vi "一体站流程自动启动.vi"(11 "参数":T1) -> ()   [LabVIEW 2016, in "PLC.lvlib"]
uses:
  PLC.lvlib
panel:
  out "s? t:f":enum16{"初始化", "采配水启动", "仪器操作", "反冲洗", "结束"}(ring)
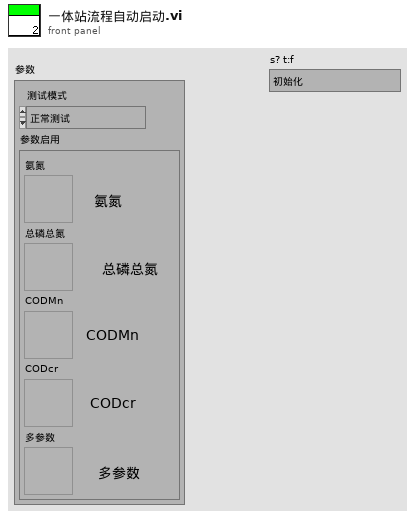
[diagram p1: front panel]
types:
  T1 = cluster{"测试模式":enum16{"正常测试", "集成干预"}, "参数启用":cluster{"氨氮":bool, "总磷总氮":bool, "CODMn":bool, "CODcr":bool, "多参数":bool}}
  T2 = cluster{"命令":string, cluster{"starting address":u16, "holding register value":u16}}
  T3 = enum16{"启动测量", "标样核查", "零点核查", "跨度核查", "空白测试", "平行样测试", "加标回收", "空白校准", "标样校准", "初始化（清洗）", "停止测试", "仪器重启", "校时", "模式设置", "测量间隔设置"}
  T4 = cluster{"时间标识":timestamp, "设备":string, "日志信息":string, "流程参数":string}
  T5 = cluster{"测量模式":enum16{"水样测量", "标样核查", "零点核查", "跨度核查", "空白测试", "加标回收", "平行样", "校零", "校标"}}
  T6 = cluster{"时间标识":timestamp, "设备":string, "日志信息":string}
  T7 = enum16{"空闲", "水样测试", "标样核查", "零点核查", "跨度核查", "空白测试", "平行样测试", "加标回收", "空白校准", "标样校准", "初始化（清洗）"}
  T8 = typedef "斯坦道多参数.lvlib/水样测试启动自定义输入参数.ctl" = cluster{"测量模式":enum16{"待机", "水样测试", "标样核查", "零点核查", "跨度核查", "空白测试", "平行样测试", "加标回收", "空白校准", "标样校准", "初始化（清洗）"}, "数据类型":string, "手动启动标记":bool, "测量时间":dbl}
  T9 = enum16{"待机", "水样测试", "标样核查", "零点核查", "跨度核查", "空白测试", "平行样测试", "加标回收", "空白校准", "标样校准", "初始化（清洗）"}
  T10 = cluster{"R0":i16, "R1":i16, "R2":i16, "R3":i16, "R4":i16, "R5":i16, "R6":i16, "R7":i16, "R8":i16, "R9":i16, "R10":i16, "R11":i16, "R12":i16, "R13":i16, "R14":i16, "R15":i16, "R16":i16, "R17":i16, "R18":i16, "R19":i16, "R20":i16, "R21":i16, "R22":i16, "R23":i16, "R24":i16, "R25":i16, "R26":i16, "R27":i16, "R28":i16, "R29":i16, "R30":i16, "R31":i16, "R32":i16, "R33":i16, "R34":i16}
  T11 = enum32{"Bad", "Idle", "Run top level", "Running"}
  T12 = cluster{"氨氮":bool, "总磷总氮":bool, "CODMn":bool, "CODcr":bool, "多参数":bool}
  T13 = cluster{"水温":dbl, "pH":dbl, "DO":dbl, "Cond":dbl, "Turb":dbl, "叶绿素":dbl, "藻密度":dbl, "蓝绿藻":dbl, "ORP":dbl, "NH3N":dbl}
  T14 = cluster{"时间标识":timestamp, "参数":string, "集成干预测试浓度值":dbl, "集成干预前测试时间":timestamp, "集成干预前测试浓度值":dbl}
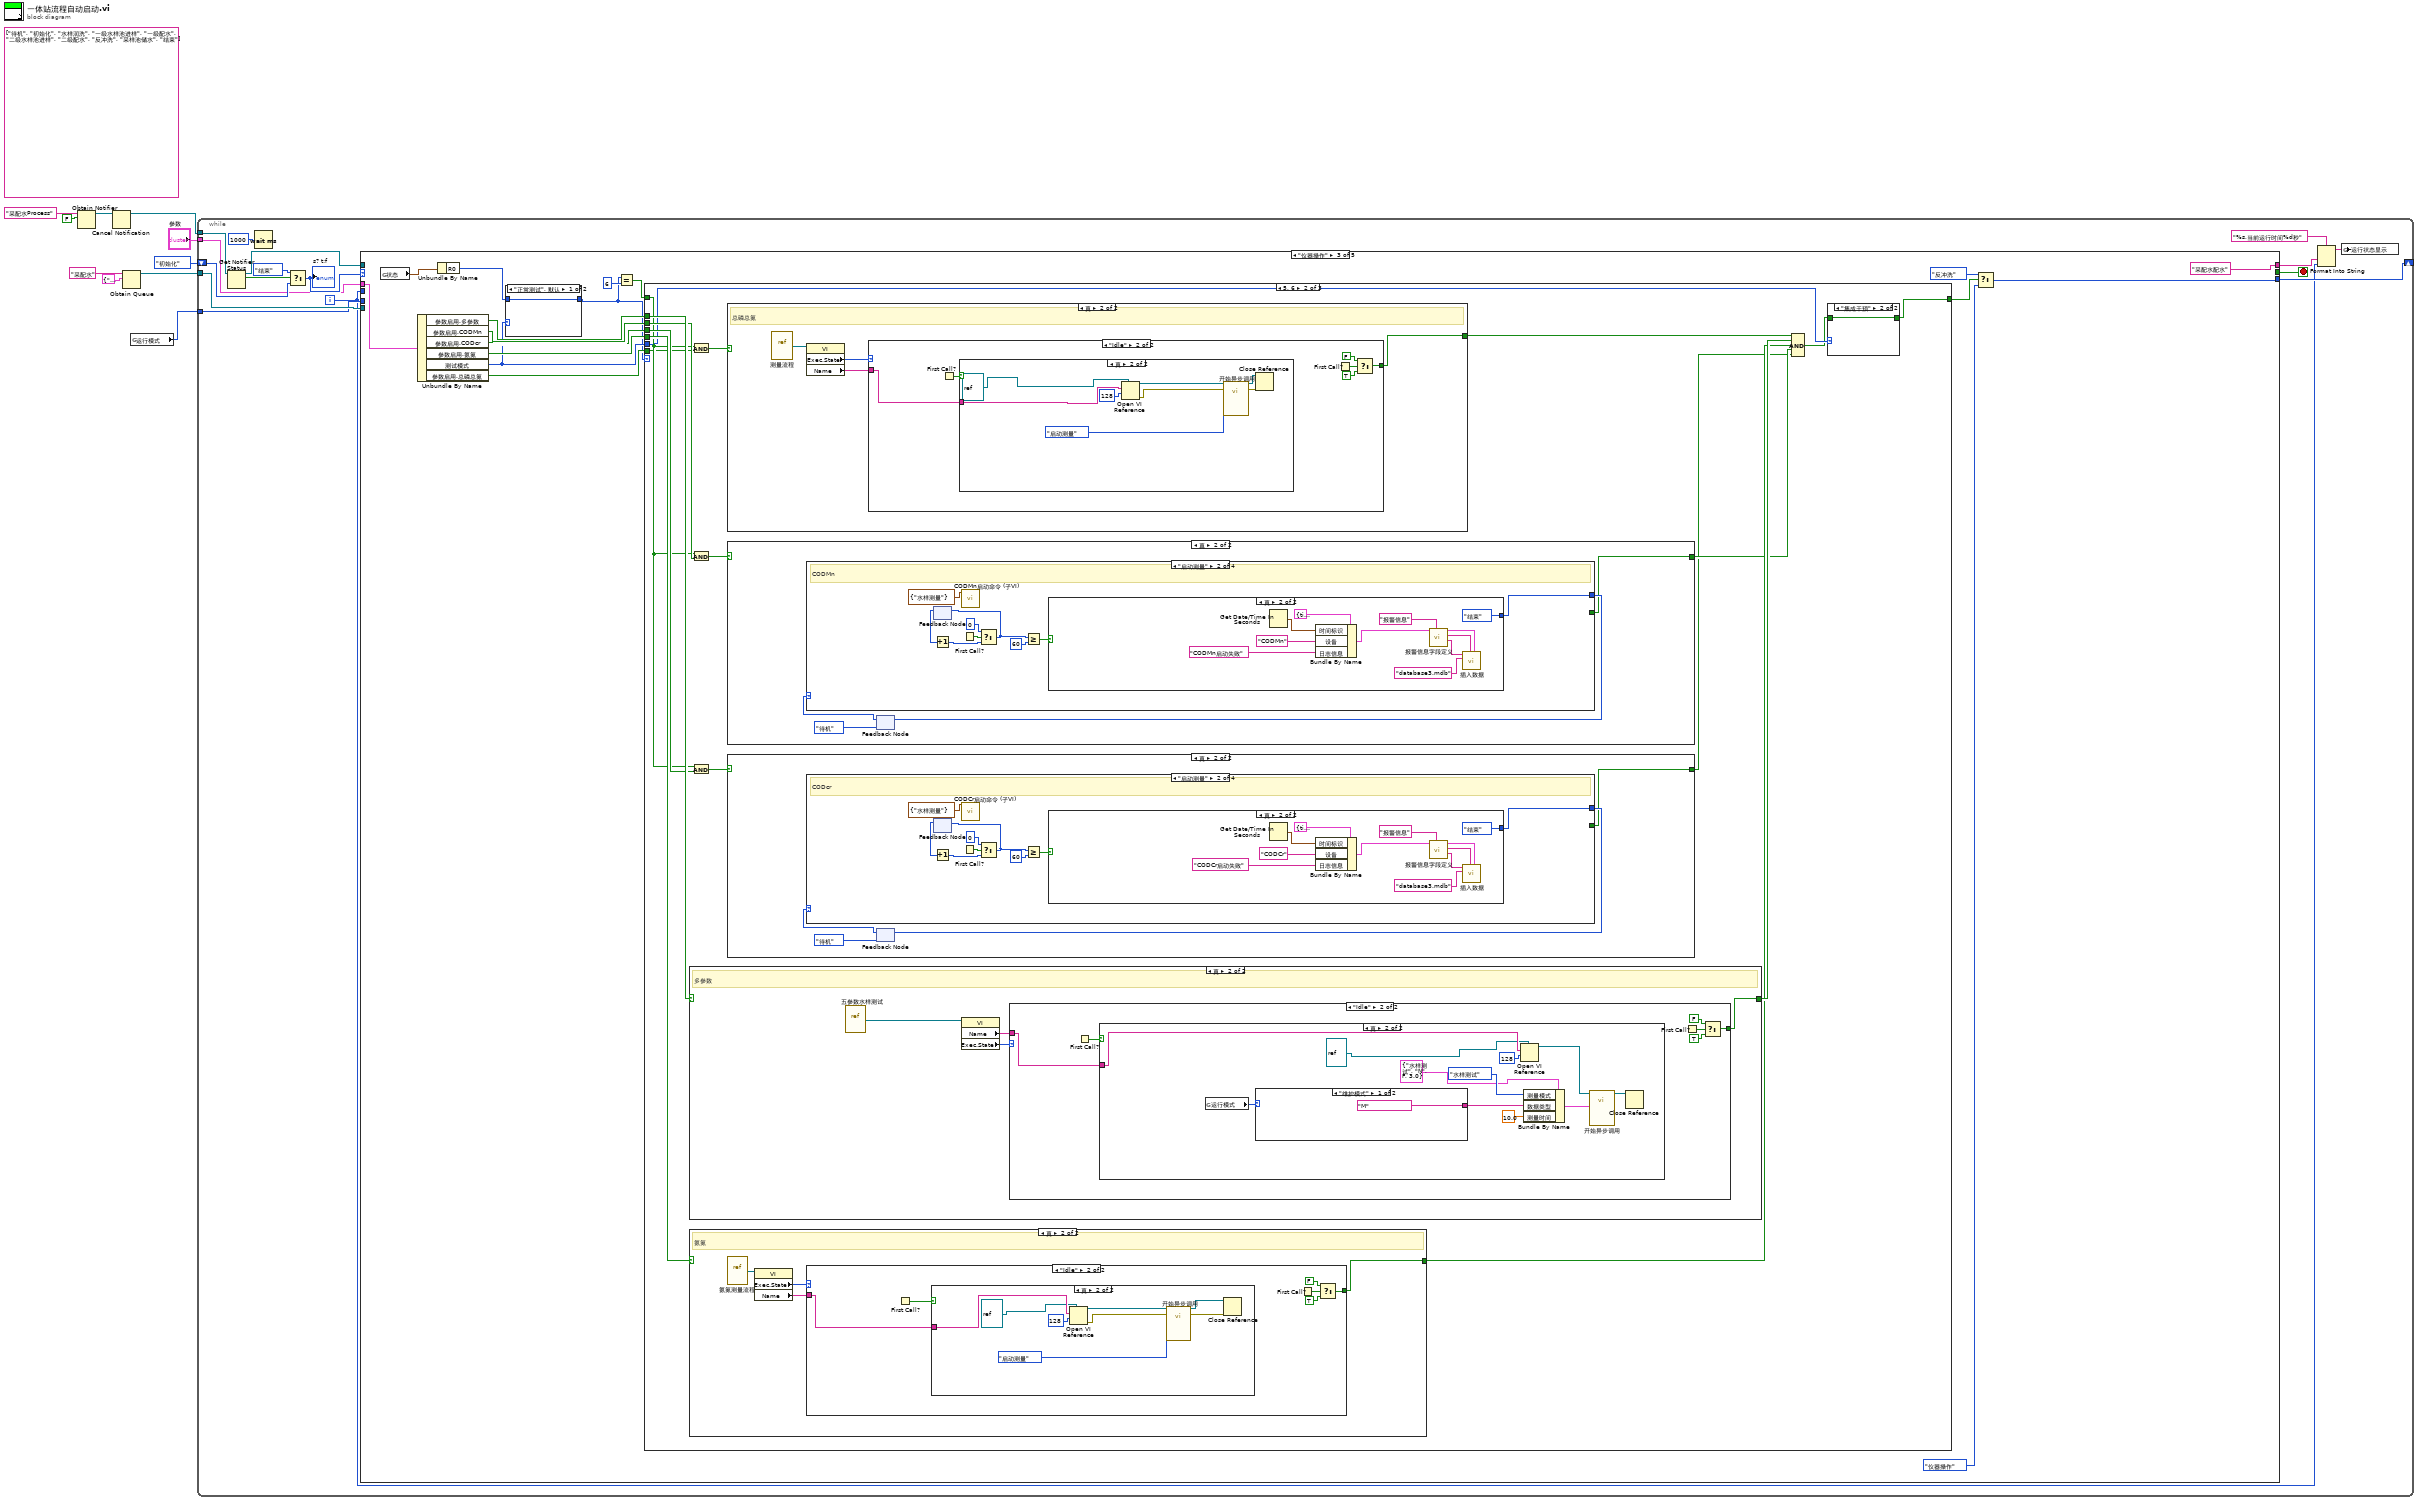
[diagram p0: block diagram]
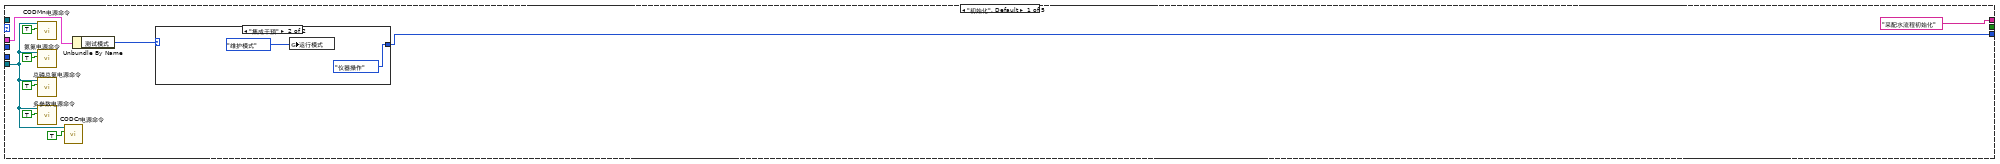
[diagram p2: hidden frame]
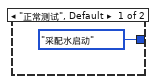
[diagram p3: hidden frame]
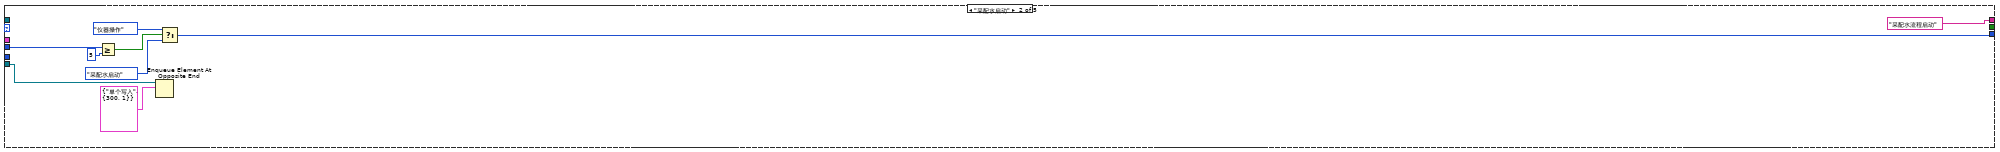
[diagram p4: hidden frame]
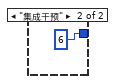
[diagram p5: hidden frame]
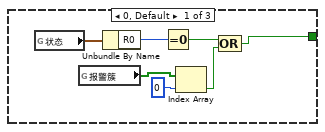
[diagram p6: hidden frame]
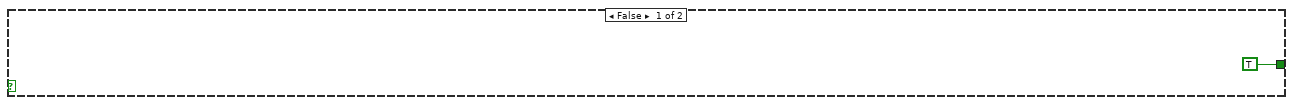
[diagram p7: hidden frame]
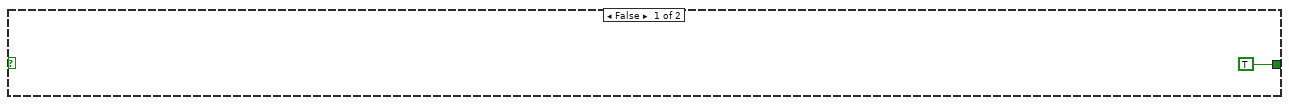
[diagram p11: hidden frame]
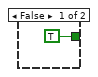
[diagram p14: hidden frame]
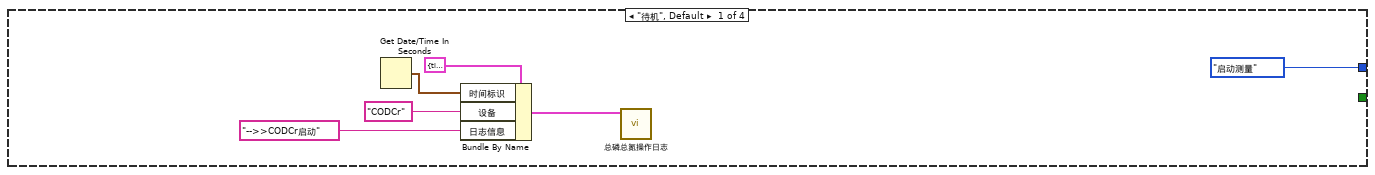
[diagram p15: hidden frame]
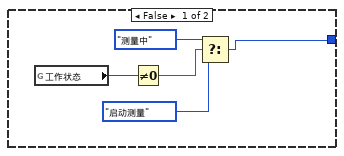
[diagram p16: hidden frame]
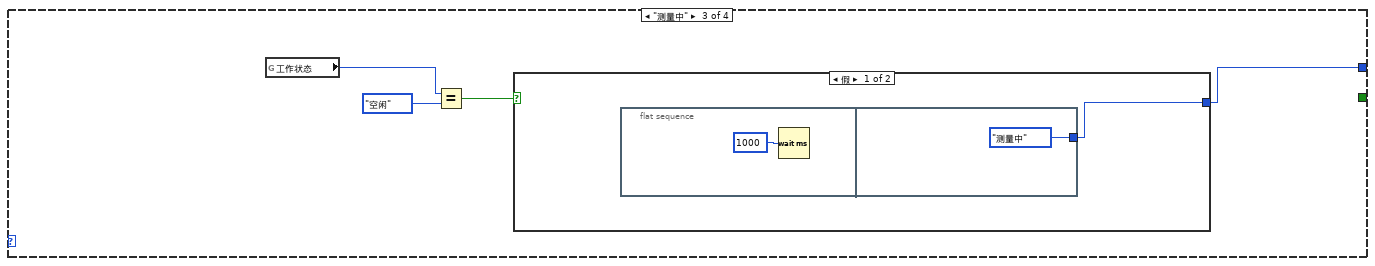
[diagram p17: hidden frame]
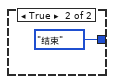
[diagram p18: hidden frame]
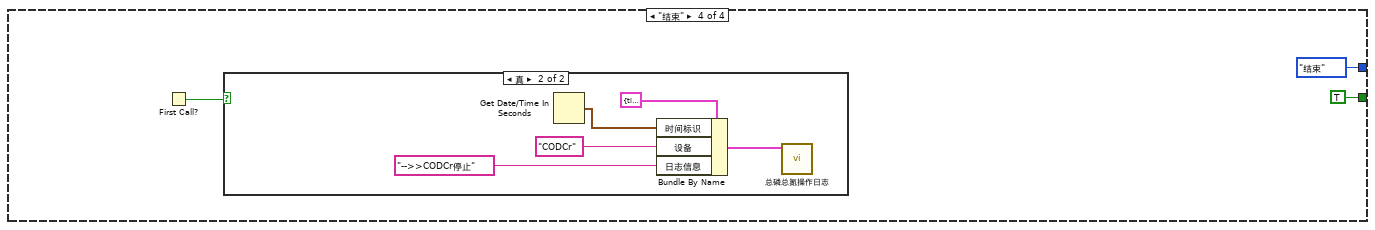
[diagram p19: hidden frame]
diagram:
  (unwired) string[][] [["待机"], ["初始化"], ["水样润洗"], ["一级水样池进样"], ["一级配水"], ["二级水样池进样"], ["二级配水"], ["反冲洗"], ["采样池储水"], ["结束"]] ("项名")
  n1 = Obtain Notifier(name (unnamed)="采配水Process" ("名称（未命名）"), notification data type=FALSE) -> (notifier out=w4:refnum<notifier>)  [unwired: 2 in, 2 out]
  n2 = Cancel Notification(0:w4) -> (8:w3:refnum<notifier>)  [unwired: 1 in, 2 out]
  n3 = Obtain Queue(name (unnamed)="采配水" ("名称（未命名）"), element data type=cluster{"命令":string, "数据":variant} {"命令"="", "数据"=variant}) -> (queue out=w7:refnum<queue>)  [unwired: 3 in, 2 out]
  n4 = global read "系统设置全局变量.vi" "运行模式"() -> (w1:enum16{"维护模式", "常规模式", "应急模式", "质控模式"})
  n5 = while {
    shift-right: [w23] -> _
    shift-left: enum16{"初始化", "采配水启动", "仪器操作", "反冲洗", "结束"}."初始化" ("枚举") -> [w19]
    tunnel: w7 -> [w26]
    tunnel: w3 -> [w22]
    tunnel: "参数" -> [w13]
    tunnel: w1 -> [w12]
    i -> [w11]
    stop <- w25 stop-if-true
    n6 = Get Notifier Status(notifier=w22) -> (notifier out=w14:refnum<notifier>, current notification=w21:bool)  [unwired: 1 in, 3 out]
    n7 = Wait (ms)(milliseconds to wait=u32 1000 ("等待时间（毫秒）")) -> ()  [unwired: 1 out]
    n8 = Select(t=enum16{"初始化", "采配水启动", "仪器操作", "反冲洗", "结束"}."结束" ("枚举"), s=w21, f=w19) -> (s? t:f=w18:enum16{"初始化", "采配水启动", "仪器操作", "反冲洗", "结束"})
    "s? t:f" <- w18
    n9 = case shown="\"仪器操作\"" w18 {
      tunnel: w26 -> [w31 w48 _ _ w438]
      tunnel: [_ _ _ _ TRUE] -> w25
      tunnel: [w30 w40 w60 w262 enum16{"初始化", "采配水启动", "仪器操作", "反冲洗", "结束"}."结束" ("枚举")] -> w23
      tunnel: ["采配水流程初始化" "采配水流程启动" "采配水配水" "等待测试完成" "采配水结束"] -> w15
      tunnel: w14 -> [_ _ _ _ w439]
      tunnel: w13 -> [w28 _ w63 w261 w435]
      tunnel: w12 -> [_ _ _ _ w434]
      tunnel: w11 -> [_ w46 _ _ _]
      frame "初始化", Default {
        n10 = call "CODMn电源命令.vi"("通电/断电"=TRUE, "队列"=w31) -> ()  [unwired: 9 in, 1 out]
        n11 = call "氨氮电源命令.vi"("通电/断电"=TRUE, "队列"=w31) -> ()  [unwired: 9 in, 1 out]
        n12 = call "总磷总氮电源命令.vi"("通电/断电"=TRUE, "队列"=w31) -> ()  [unwired: 9 in, 1 out]
        n13 = call "多参数电源命令.vi"("通电/断电"=TRUE, "队列"=w31) -> ()  [unwired: 9 in, 1 out]
        n14 = call "CODCr电源命令.vi"("通电/断电"=TRUE, "队列"=w31) -> ()  [unwired: 9 in, 1 out]
        n15 = Unbundle By Name(w28) -> ("测试模式"=w27:enum16{"正常测试", "集成干预"})
        n16 = case shown="\"集成干预\"" w27 {
          tunnel: [enum16{"初始化", "采配水启动", "仪器操作", "反冲洗", "结束"}."采配水启动" ("枚举") enum16{"初始化", "采配水启动", "仪器操作", "反冲洗", "结束"}."仪器操作" ("枚举")] -> w30
          frame "正常测试", Default {
          }
          frame "集成干预" {
            n17 = global write "系统设置全局变量.vi" "运行模式"(enum16{"维护模式", "常规模式", "应急模式", "质控模式"}."维护模式" ("运行模式")) -> ()
          }
        }
      }
      frame "采配水启动" {
        n18 = Greater Or Equal?(x=w46, y=5) -> (x >= y?=w43:bool)
        n19 = Enqueue Element At Opposite End(queue=w48, element=T2 {"命令"="单个写入", {"starting address"=300, "holding register value"=1}} ("元素")) -> ()  [unwired: 2 in, 3 out]
        n20 = Select(t=enum16{"初始化", "采配水启动", "仪器操作", "反冲洗", "结束"}."仪器操作" ("枚举"), s=w43, f=enum16{"初始化", "采配水启动", "仪器操作", "反冲洗", "结束"}."采配水启动" ("枚举")) -> (s? t:f=w40:enum16{"初始化", "采配水启动", "仪器操作", "反冲洗", "结束"})
      }
      frame "仪器操作" {
        n21 = global read "采配水全局变量.vi" "状态"() -> (w65:T10)
        n22 = Unbundle By Name(w63) -> ("参数启用.多参数"=w58:bool, "参数启用.CODMn"=w57:bool, "参数启用.CODcr"=w56:bool, "参数启用.氨氮"=w55:bool, "测试模式"=w53:enum16{"正常测试", "集成干预"}, "参数启用.总磷总氮"=w52:bool)
        n23 = Unbundle By Name(w65) -> ("R0"=w54:i16)
        n24 = case shown="\"正常测试\", 默认" w53 {
          tunnel: w54 -> [w66 _]
          tunnel: [w66 i16 6 ("R0")] -> w50
          frame "正常测试", Default {
          }
          frame "集成干预" {
          }
        }
        n25 = Equal?(x=w50, y=i16 6) -> (x = y?=w49:bool)
        n26 = case shown="5, 6" w50 {
          tunnel: [w69 w79 TRUE] -> w62
          tunnel: w58 -> [_ w91 _]
          tunnel: w57 -> [_ w90 _]
          tunnel: w56 -> [_ w87 _]
          tunnel: w55 -> [_ w86 _]
          tunnel: w49 -> [_ w78 _]
          tunnel: w53 -> [_ w81 _]
          tunnel: w52 -> [_ w77 _]
          frame 0, Default {
            n27 = global read "采配水全局变量.vi" "状态"() -> (w72:T10)
            n28 = global read "采配水全局变量.vi" "报警簇"() -> (w73:bool[])
            n29 = Unbundle By Name(w72) -> ("R0"=w71:i16)
            n30 = Equal To 0?(x=w71) -> (x = 0?=w74:bool)
            n31 = Index Array(array=w73, index=0 ("索引")) -> (element=w68:bool)
            n32 = Compound Arithmetic op=OR ("复合运算")(w74, w68) -> (w69:bool)
          }
          frame 5, 6 {
            n33 = case shown="真" w91 {
              tunnel: [TRUE ("t") w235] -> w85
              frame False {
              }
              frame True {
                # "多参数"
                n34 = vi-ref "五参数水样测试.vi"() -> (w237:refnum<vi>)
                n35 = property class="VI"(reference=w237) -> ("Name"=w236:string, "Exec.State"=w238:T11)  [unwired: 1 in, 2 out]
                n36 = case shown="\"Idle\"" w238 {
                  tunnel: w236 -> [_ w244]
                  tunnel: [_ w239] -> w235
                  frame "Bad", Default {
                  }
                  frame "Idle" {
                    n37 = First Call?() -> (First Call?: T/F=w243:bool)
                    n38 = case shown="真" w243 {
                      tunnel: w244 -> [_ w253]
                      frame False {
                      }
                      frame True {
                        n39 = global read "系统设置全局变量.vi" "运行模式"() -> (w250:enum16{"维护模式", "常规模式", "应急模式", "质控模式"})
                        n40 = case shown="\"维护模式\"" w250 {
                          tunnel: ["M" ("数据标记表") "N" ("数据标记表")] -> w249
                          frame "维护模式" {
                          }
                          frame "常规模式", Default {
                          }
                        }
                        n41 = Open VI Reference(type specifier VI Refnum (for type only)=refnum<vi> refnum, vi path=w253, options=128 ("选项")) -> (vi reference=w252:refnum<vi>)  [unwired: 3 in, 1 out]
                        n42 = Bundle By Name(cluster=T8 {"测量模式"=enum."水样测试", "数据类型"="N", "手动启动标记"=FALSE, "测量时间"=3.0} ("启动参数"), "测量模式"=T9."水样测试", "数据类型"=w249, "测量时间"=10.0) -> (w245:T8)
                        n43 = call-by-ref "开始异步调用"(reference=w252, "启动参数"=w245) -> (reference out=w251:refnum<vi>)  [unwired: 12 in, 1 out]
                        n44 = Close Reference(reference=w251) -> ()  [unwired: 1 in, 1 out]
                      }
                    }
                    n45 = First Call?() -> (First Call?: T/F=w242:bool)
                    n46 = Select(t=FALSE, s=w242, f=TRUE) -> (s? t:f=w239:bool)
                  }
                }
              }
            }
            n47 = case "条件结构" shown="真" w86 {
              tunnel: [TRUE ("t") w113] -> w84
              frame False {
              }
              frame True {
                # "氨氮"
                n48 = vi-ref "氨氮测量流程.vi"() -> (w116:refnum<vi>)
                n49 = property class="VI"(reference=w116) -> ("Exec.State"=w115:T11, "Name"=w114:string)  [unwired: 1 in, 2 out]
                n50 = case shown="\"Idle\"" w115 {
                  tunnel: w114 -> [_ w122]
                  tunnel: [_ w117] -> w113
                  frame "Bad", Default {
                  }
                  frame "Idle" {
                    n51 = First Call?() -> (First Call?: T/F=w121:bool)
                    n52 = case shown="真" w121 {
                      tunnel: w122 -> [_ w127]
                      frame False {
                      }
                      frame True {
                        n53 = Open VI Reference(type specifier VI Refnum (for type only)=refnum<vi> refnum, vi path=w127, options=128 ("选项")) -> (vi reference=w125:refnum<vi>, error out=w128:errorcluster)  [unwired: 3 in]
                        n54 = call-by-ref "开始异步调用"(reference=w125, error in=w128, "控制命令"=T3."启动测量") -> (reference out=w129:refnum<vi>, error out=w130:errorcluster)  [unwired: 11 in]
                        n55 = Close Reference(reference=w129, error in (no error)=w130) -> ()  [unwired: 1 out]
                      }
                    }
                    n56 = First Call?() -> (First Call?: T/F=w120:bool)
                    n57 = Select(t=FALSE, s=w120, f=TRUE) -> (s? t:f=w117:bool)
                  }
                }
              }
            }
            n58 = And(x=w78, y=w77) -> (x .and. y?=w76:bool)
            n59 = And(x=w78, y=w90) -> (x .and. y?=w89:bool)
            n60 = And(x=w78, y=w87) -> (x .and. y?=w88:bool)
            n61 = case "条件结构" shown="真" w76 {
              tunnel: [TRUE ("t") w93] -> w75
              frame False {
              }
              frame True {
                # "总磷总氮"
                n62 = vi-ref "测量流程.vi"() -> (w96:refnum<vi>)
                n63 = property class="VI"(reference=w96) -> ("Exec.State"=w95:T11, "Name"=w94:string)  [unwired: 1 in, 2 out]
                n64 = case shown="\"Idle\"" w95 {
                  tunnel: w94 -> [_ w102]
                  tunnel: [_ w97] -> w93
                  frame "Bad", Default {
                  }
                  frame "Idle" {
                    n65 = First Call?() -> (First Call?: T/F=w101:bool)
                    n66 = case shown="真" w101 {
                      tunnel: w102 -> [_ w107]
                      frame False {
                      }
                      frame True {
                        n67 = Open VI Reference(type specifier VI Refnum (for type only)=refnum<vi> refnum, vi path=w107, options=128 ("选项")) -> (vi reference=w105:refnum<vi>, error out=w108:errorcluster)  [unwired: 3 in]
                        n68 = call-by-ref "开始异步调用"(reference=w105, error in=w108, "控制命令"=T3."启动测量") -> (reference out=w109:refnum<vi>, error out=w110:errorcluster)  [unwired: 11 in]
                        n69 = Close Reference(reference=w109, error in (no error)=w110) -> ()  [unwired: 1 out]
                      }
                    }
                    n70 = First Call?() -> (First Call?: T/F=w100:bool)
                    n71 = Select(t=FALSE, s=w100, f=TRUE) -> (s? t:f=w97:bool)
                  }
                }
              }
            }
            n72 = case shown="真" w89 {
              tunnel: [TRUE w184] -> w83
              frame False {
              }
              frame True {
                n73 = feedback #1(enum16{"待机", "启动测量", "测量中", "结束"}."待机") -> (w186:enum16{"待机", "启动测量", "测量中", "结束"})
                n74 = case shown="\"启动测量\"" w186 {
                  tunnel: [enum16{"待机", "启动测量", "测量中", "结束"}."启动测量" w202 w221 enum16{"待机", "启动测量", "测量中", "结束"}."结束"] -> w185
                  tunnel: [_ _ _ TRUE] -> w184
                  frame "待机", Default {
                    n75 = Get Date/Time In Seconds() -> (seconds since 1Jan1904=w192:timestamp)
                    n76 = Bundle By Name(cluster=T4 {"时间标识"=timestamp(0 s since 1904-01-01), "设备"="", "日志信息"="", "流程参数"=""} ("data in"), "时间标识"=w192, "设备"="CODMn", "日志信息"="-->>CODMn启动") -> (w188:T4)
                    n77 = call "总磷总氮操作日志.vi"("data in"=w188) -> ()  [unwired: 11 in]
                  }
                  frame "启动测量" {
                    # "CODMn"
                    n78 = feedback #2() -> (w198:i32)  [unwired: 1 in]
                    n79 = Increment(x=w198) -> (x+1=w199:i32)
                    n80 = First Call?() -> (First Call?: T/F=w197:bool)
                    n81 = call "CODMn启动命令 (子VI).vi"("启动测量模式"=T5 {"测量模式"=enum."水样测量"}) -> ()  [unwired: 11 in]
                    n82 = Select(t=0, s=w197, f=w199) -> (s? t:f=w200:i32)
                    n83 = feedback-in #2(w200) -> ()
                    n84 = Greater Or Equal?(x=w200, y=60) -> (x >= y?=w195:bool)
                    n85 = case shown="真" w195 {
                      tunnel: [w204 enum16{"待机", "启动测量", "测量中", "结束"}."结束"] -> w202
                      frame False {
                        n86 = global read "运行时序全局变量.vi" "多列列表框"() -> (w203:i32)
                        n87 = Not Equal To 0?(x=w203) -> (x != 0?=w205:bool)
                        n88 = Select(t=enum16{"待机", "启动测量", "测量中", "结束"}."测量中", s=w205, f=enum16{"待机", "启动测量", "测量中", "结束"}."启动测量") -> (s? t:f=w204:enum16{"待机", "启动测量", "测量中", "结束"})
                      }
                      frame True {
                        n89 = Get Date/Time In Seconds() -> (seconds since 1Jan1904=w214:timestamp)
                        n90 = Bundle By Name(cluster=T6 {"时间标识"=timestamp(0 s since 1904-01-01), "设备"="", "日志信息"=""} ("data in"), "时间标识"=w214, "设备"="CODMn", "日志信息"="CODMn启动失败") -> (w208:T6)
                        n91 = call "报警信息字段定义.vi"("table输入"="报警信息", "data in"=w208) -> ("table输出"=w211:string, "columns"=w212:string[], "data out"=w213:T6)  [unwired: 7 in]
                        n92 = call "插入数据.vi"("data"=w213, "columns"=w212, "database"="database3.mdb", "table"=w211) -> ()  [unwired: 7 in, 1 out]
                      }
                    }
                  }
                  frame "测量中" {
                    n93 = global read "运行时序全局变量.vi" "多列列表框"() -> (w220:i32)
                    n94 = Equal To 0?(x=w220) -> (x = 0?=w219:bool)
                    n95 = case shown="假" w219 {
                      tunnel: [w222 enum16{"待机", "启动测量", "测量中", "结束"}."结束"] -> w221
                      frame False {
                        n96 = flat-sequence {
                          tunnel: [enum16{"待机", "启动测量", "测量中", "结束"}."测量中"] -> w222
                          frame #0 {
                            n97 = Wait (ms)(milliseconds to wait=u32 1000 ("等待时间（毫秒）")) -> ()  [unwired: 1 out]
                          }
                          frame #1 {
                          }
                        }
                      }
                      frame True {
                      }
                    }
                  }
                  frame "结束" {
                    n98 = First Call?() -> (First Call?: T/F=w226:bool)
                    n99 = case shown="真" w226 {
                      frame False {
                      }
                      frame True {
                        n100 = Get Date/Time In Seconds() -> (seconds since 1Jan1904=w233:timestamp)
                        n101 = Bundle By Name(cluster=T4 {"时间标识"=timestamp(0 s since 1904-01-01), "设备"="", "日志信息"="", "流程参数"=""} ("data in"), "时间标识"=w233, "设备"="CODMn", "日志信息"="-->>CODMn停止") -> (w229:T4)
                        n102 = call "总磷总氮操作日志.vi"("data in"=w229) -> ()  [unwired: 11 in]
                      }
                    }
                  }
                }
                n103 = feedback-in #1(w185) -> ()
              }
            }
            n104 = case shown="真" w88 {
              tunnel: [TRUE w132] -> w82
              frame False {
              }
              frame True {
                n105 = feedback #3(enum16{"待机", "启动测量", "测量中", "结束"}."待机") -> (w134:enum16{"待机", "启动测量", "测量中", "结束"})
                n106 = case shown="\"启动测量\"" w134 {
                  tunnel: [enum16{"待机", "启动测量", "测量中", "结束"}."启动测量" w150 w170 enum16{"待机", "启动测量", "测量中", "结束"}."结束"] -> w133
                  tunnel: [_ _ _ TRUE] -> w132
                  frame "待机", Default {
                    n107 = Get Date/Time In Seconds() -> (seconds since 1Jan1904=w140:timestamp)
                    n108 = Bundle By Name(cluster=T4 {"时间标识"=timestamp(0 s since 1904-01-01), "设备"="", "日志信息"="", "流程参数"=""} ("data in"), "时间标识"=w140, "设备"="CODCr", "日志信息"="-->>CODCr启动") -> (w136:T4)
                    n109 = call "总磷总氮操作日志.vi"("data in"=w136) -> ()  [unwired: 11 in]
                  }
                  frame "启动测量" {
                    # "CODcr"
                    n110 = feedback #4() -> (w146:i32)  [unwired: 1 in]
                    n111 = Increment(x=w146) -> (x+1=w147:i32)
                    n112 = First Call?() -> (First Call?: T/F=w145:bool)
                    n113 = call "CODCr启动命令 (子VI).vi"("启动测量模式"=T5 {"测量模式"=enum."水样测量"}) -> ()  [unwired: 11 in]
                    n114 = Select(t=0, s=w145, f=w147) -> (s? t:f=w148:i32)
                    n115 = feedback-in #4(w148) -> ()
                    n116 = Greater Or Equal?(x=w148, y=60) -> (x >= y?=w143:bool)
                    n117 = case shown="真" w143 {
                      tunnel: [w151 enum16{"待机", "启动测量", "测量中", "结束"}."结束"] -> w150
                      frame False {
                        n118 = global read "CODcr全局变量.vi" "工作状态"() -> (w152:T7)
                        n119 = Not Equal To 0?(x=w152) -> (x != 0?=w153:bool)
                        n120 = Select(t=enum16{"待机", "启动测量", "测量中", "结束"}."测量中", s=w153, f=enum16{"待机", "启动测量", "测量中", "结束"}."启动测量") -> (s? t:f=w151:enum16{"待机", "启动测量", "测量中", "结束"})
                      }
                      frame True {
                        n121 = Get Date/Time In Seconds() -> (seconds since 1Jan1904=w162:timestamp)
                        n122 = Bundle By Name(cluster=T6 {"时间标识"=timestamp(0 s since 1904-01-01), "设备"="", "日志信息"=""} ("data in"), "时间标识"=w162, "设备"="CODCr", "日志信息"="CODCr启动失败") -> (w156:T6)
                        n123 = call "报警信息字段定义.vi"("table输入"="报警信息", "data in"=w156) -> ("table输出"=w159:string, "columns"=w160:string[], "data out"=w161:T6)  [unwired: 7 in]
                        n124 = call "插入数据.vi"("data"=w161, "columns"=w160, "database"="database3.mdb", "table"=w159) -> ()  [unwired: 7 in, 1 out]
                      }
                    }
                  }
                  frame "测量中" {
                    n125 = global read "CODcr全局变量.vi" "工作状态"() -> (w169:T7)
                    n126 = Equal?(x=w169, y=T7."空闲" ("工作状态")) -> (x = y?=w168:bool)
                    n127 = case shown="假" w168 {
                      tunnel: [w171 enum16{"待机", "启动测量", "测量中", "结束"}."结束"] -> w170
                      frame False {
                        n128 = flat-sequence {
                          tunnel: [enum16{"待机", "启动测量", "测量中", "结束"}."测量中"] -> w171
                          frame #0 {
                            n129 = Wait (ms)(milliseconds to wait=u32 1000 ("等待时间（毫秒）")) -> ()  [unwired: 1 out]
                          }
                          frame #1 {
                          }
                        }
                      }
                      frame True {
                      }
                    }
                  }
                  frame "结束" {
                    n130 = First Call?() -> (First Call?: T/F=w175:bool)
                    n131 = case shown="真" w175 {
                      frame False {
                      }
                      frame True {
                        n132 = Get Date/Time In Seconds() -> (seconds since 1Jan1904=w182:timestamp)
                        n133 = Bundle By Name(cluster=T4 {"时间标识"=timestamp(0 s since 1904-01-01), "设备"="", "日志信息"="", "流程参数"=""} ("data in"), "时间标识"=w182, "设备"="CODCr", "日志信息"="-->>CODCr停止") -> (w178:T4)
                        n134 = call "总磷总氮操作日志.vi"("data in"=w178) -> ()  [unwired: 11 in]
                      }
                    }
                  }
                }
                n135 = feedback-in #3(w133) -> ()
              }
            }
            n136 = Compound Arithmetic op=AND ("复合运算")(w75, w85, w84, w83, w82) -> (w80:bool)
            n137 = case shown="\"集成干预\"" w81 {
              tunnel: w80 -> [_ w111]
              tunnel: [_ w111] -> w79
              frame "正常测试", Default {
              }
              frame "集成干预" {
              }
            }
          }
          frame 7..9 {
          }
        }
        n138 = Select(t=enum16{"初始化", "采配水启动", "仪器操作", "反冲洗", "结束"}."反冲洗" ("枚举"), s=w62, f=enum16{"初始化", "采配水启动", "仪器操作", "反冲洗", "结束"}."仪器操作" ("枚举")) -> (s? t:f=w60:enum16{"初始化", "采配水启动", "仪器操作", "反冲洗", "结束"})
      }
      frame "反冲洗" {
        n139 = First Call?() -> (First Call?: T/F=w259:bool)
        n140 = case shown="真" w259 {
          tunnel: w261 -> [_ w270]
          frame False {
          }
          frame True {
            n141 = Unbundle By Name(w270) -> ("测试模式"=w269:enum16{"正常测试", "集成干预"}, "参数启用"=w268:T12)
            n142 = case shown="\"正常测试\", 默认" w269 {
              tunnel: w268 -> [w273 w365]
              frame "正常测试", Default {
                n143 = global read "系统设置全局变量.vi" "运行模式"() -> (w271:enum16{"维护模式", "常规模式", "应急模式", "质控模式"})
                n144 = global read "采配水全局变量.vi" "报警簇"() -> (w278:bool[])
                n145 = case shown="\"维护模式\"" w271 {
                  tunnel: ["M" ("table") "N" ("table")] -> w272
                  frame "维护模式" {
                  }
                  frame "常规模式", Default {
                  }
                }
                n146 = Index Array(array=w278, index #1=0 ("索引"), index #2=11 ("索引")) -> (element #1=w275:bool, element #2=w274:bool)
                n147 = case shown="真" w275 {
                  tunnel: w274 -> [w284 _]
                  tunnel: w273 -> [w283 w297]
                  tunnel: w272 -> [w281 w291]
                  frame False {
                    n148 = Unbundle By Name(w283) -> ("氨氮"=w282:bool)
                    n149 = case shown="真" w284 {
                      tunnel: w282 -> [_ w286]
                      tunnel: w281 -> [_ w285]
                      frame False {
                      }
                      frame True {
                        n150 = case shown="真" w286 {
                          tunnel: w285 -> [_ w287]
                          tunnel: [_ w288] -> _
                          frame False {
                          }
                          frame True {
                            n151 = call "取水点无水样数据存储.vi"("数据标识"="lw", "数据类型"=w287, "table"="氨氮") -> ("error out"=w288:errorcluster)  [unwired: 8 in]
                          }
                        }
                      }
                    }
                  }
                  frame True {
                    n152 = Unbundle By Name(w297) -> ("氨氮"=w296:bool, "CODMn"=w295:bool, "CODcr"=w294:bool, "多参数"=w293:bool, "总磷总氮"=w292:bool)
                    n153 = case shown="真" w296 {
                      tunnel: w291 -> [_ w357]
                      tunnel: [_ w358] -> _
                      frame False {
                      }
                      frame True {
                        n154 = call "取水点无水样数据存储.vi"("数据标识"="Z", "数据类型"=w357, "table"="氨氮") -> ("error out"=w358:errorcluster)  [unwired: 8 in]
                      }
                    }
                    n155 = case shown="真" w295 {
                      tunnel: w291 -> [_ w354]
                      tunnel: [_ w353] -> _
                      frame False {
                      }
                      frame True {
                        n156 = call "取水点无水样数据存储.vi"("数据标识"="Z", "数据类型"=w354, "table"="CODMn") -> ("error out"=w353:errorcluster)  [unwired: 8 in]
                      }
                    }
                    n157 = case shown="真" w294 {
                      tunnel: w291 -> [_ w350]
                      tunnel: [_ w349] -> _
                      frame False {
                      }
                      frame True {
                        n158 = call "取水点无水样数据存储.vi"("数据标识"="Z", "数据类型"=w350, "table"="CODCr") -> ("error out"=w349:errorcluster)  [unwired: 8 in]
                      }
                    }
                    n159 = case shown="真" w292 {
                      tunnel: w291 -> [_ w299]
                      tunnel: [_ w298] -> _
                      frame False {
                      }
                      frame True {
                        n160 = call "取水点无水样数据存储.vi"("数据标识"="Z", "数据类型"=w299, "table"="总氮") -> ("error out"=w300:errorcluster)  [unwired: 8 in]
                        n161 = call "取水点无水样数据存储.vi"("error in (no error)"=w300, "数据标识"="Z", "数据类型"=w299, "table"="总磷") -> ("error out"=w298:errorcluster)  [unwired: 7 in]
                      }
                    }
                    n162 = case shown="真" w293 {
                      tunnel: w291 -> [_ w305]
                      frame False {
                      }
                      frame True {
                        n163 = global read "多参数全局变量.vi" "传感器通道号"() -> (w320:T13)
                        n164 = Unbundle By Name(w320) -> ("水温"=w319:dbl, "pH"=w318:dbl, "DO"=w317:dbl, "Cond"=w316:dbl, "Turb"=w315:dbl, "叶绿素"=w314:dbl, "藻密度"=w313:dbl)
                        n165 = Not Equal To 0?(x=w319) -> (x != 0?=w312:bool)
                        n166 = Not Equal To 0?(x=w318) -> (x != 0?=w311:bool)
                        n167 = Not Equal To 0?(x=w317) -> (x != 0?=w310:bool)
                        n168 = Not Equal To 0?(x=w316) -> (x != 0?=w309:bool)
                        n169 = Not Equal To 0?(x=w315) -> (x != 0?=w308:bool)
                        n170 = Not Equal To 0?(x=w314) -> (x != 0?=w307:bool)
                        n171 = Not Equal To 0?(x=w313) -> (x != 0?=w306:bool)
                        n172 = case shown="真" w312 {
                          tunnel: w305 -> [_ w346]
                          tunnel: [_ w345] -> _
                          frame False {
                          }
                          frame True {
                            n173 = call "取水点无水样数据存储.vi"("数据标识"="Z", "数据类型"=w346, "table"="水温") -> ("error out"=w345:errorcluster)  [unwired: 8 in]
                          }
                        }
                        n174 = case shown="真" w311 {
                          tunnel: w305 -> [_ w342]
                          tunnel: [_ w341] -> _
                          frame False {
                          }
                          frame True {
                            n175 = call "取水点无水样数据存储.vi"("数据标识"="Z", "数据类型"=w342, "table"="pH") -> ("error out"=w341:errorcluster)  [unwired: 8 in]
                          }
                        }
                        n176 = case shown="真" w310 {
                          tunnel: w305 -> [_ w338]
                          tunnel: [_ w337] -> _
                          frame False {
                          }
                          frame True {
                            n177 = call "取水点无水样数据存储.vi"("数据标识"="Z", "数据类型"=w338, "table"="DO") -> ("error out"=w337:errorcluster)  [unwired: 8 in]
                          }
                        }
                        n178 = case shown="真" w308 {
                          tunnel: w305 -> [_ w330]
                          tunnel: [_ w329] -> _
                          frame False {
                          }
                          frame True {
                            n179 = call "取水点无水样数据存储.vi"("数据标识"="Z", "数据类型"=w330, "table"="浊度") -> ("error out"=w329:errorcluster)  [unwired: 8 in]
                          }
                        }
                        n180 = case shown="真" w309 {
                          tunnel: w305 -> [_ w334]
                          tunnel: [_ w333] -> _
                          frame False {
                          }
                          frame True {
                            n181 = call "取水点无水样数据存储.vi"("数据标识"="Z", "数据类型"=w334, "table"="比电导率") -> ("error out"=w333:errorcluster)  [unwired: 8 in]
                          }
                        }
                        n182 = case shown="真" w307 {
                          tunnel: w305 -> [_ w326]
                          tunnel: [_ w325] -> _
                          frame False {
                          }
                          frame True {
                            n183 = call "取水点无水样数据存储.vi"("数据标识"="Z", "数据类型"=w326, "table"="叶绿素") -> ("error out"=w325:errorcluster)  [unwired: 8 in]
                          }
                        }
                        n184 = case shown="真" w306 {
                          tunnel: w305 -> [_ w322]
                          tunnel: [_ w321] -> _
                          frame False {
                          }
                          frame True {
                            n185 = call "取水点无水样数据存储.vi"("数据标识"="Z", "数据类型"=w322, "table"="藻密度") -> ("error out"=w321:errorcluster)  [unwired: 8 in]
                          }
                        }
                      }
                    }
                  }
                }
              }
              frame "集成干预" {
                n186 = Unbundle By Name(w365) -> ("氨氮"=w364:bool, "CODMn"=w363:bool, "CODcr"=w362:bool, "多参数"=w361:bool)
                n187 = case shown="真" w364 {
                  frame False {
                  }
                  frame True {
                    n188 = call "获取最近两组水样测试数据.vi"("table"="氨氮") -> ("error out"=w431:errorcluster, "存储变量"=w432:T14)  [unwired: 9 in]
                    n189 = call "集成干预测试数据存储.vi"("error in (no error)"=w431, "存储变量"=w432) -> ("error out"=w427:errorcluster)  [unwired: 9 in]
                    n190 = call "获取最近两组水样测试数据.vi"("error in (no error)"=w427, "table"="总磷") -> ("error out"=w430:errorcluster, "存储变量"=w429:T14)  [unwired: 8 in]
                    n191 = call "集成干预测试数据存储.vi"("error in (no error)"=w430, "存储变量"=w429) -> ()  [unwired: 9 in, 1 out]
                  }
                }
                n192 = case shown="真" w363 {
                  frame False {
                  }
                  frame True {
                    n193 = call "获取最近两组水样测试数据.vi"("table"="CODMn") -> ("error out"=w424:errorcluster, "存储变量"=w425:T14)  [unwired: 9 in]
                    n194 = call "集成干预测试数据存储.vi"("error in (no error)"=w424, "存储变量"=w425) -> ()  [unwired: 9 in, 1 out]
                  }
                }
                n195 = case shown="真" w362 {
                  frame False {
                  }
                  frame True {
                    n196 = call "获取最近两组水样测试数据.vi"("table"="CODCr") -> ("error out"=w421:errorcluster, "存储变量"=w422:T14)  [unwired: 9 in]
                    n197 = call "集成干预测试数据存储.vi"("error in (no error)"=w421, "存储变量"=w422) -> ()  [unwired: 9 in, 1 out]
                  }
                }
                n198 = case shown="真" w361 {
                  frame False {
                  }
                  frame True {
                    n199 = global read "多参数全局变量.vi" "传感器通道号"() -> (w386:T13)
                    n200 = Unbundle By Name(w386) -> ("水温"=w385:dbl, "pH"=w382:dbl, "DO"=w379:dbl, "Cond"=w376:dbl, "Turb"=w374:dbl, "叶绿素"=w373:dbl, "藻密度"=w372:dbl)
                    n201 = Not Equal To 0?(x=w385) -> (x != 0?=w384:bool)
                    n202 = Not Equal To 0?(x=w382) -> (x != 0?=w381:bool)
                    n203 = case shown="真" w384 {
                      tunnel: [_ w417] -> w383
                      frame False {
                      }
                      frame True {
                        n204 = call "获取最近两组水样测试数据.vi"("table"="水温") -> ("error out"=w420:errorcluster, "存储变量"=w419:T14)  [unwired: 9 in]
                        n205 = call "集成干预测试数据存储.vi"("error in (no error)"=w420, "存储变量"=w419) -> ("error out"=w417:errorcluster)  [unwired: 9 in]
                      }
                    }
                    n206 = Not Equal To 0?(x=w372) -> (x != 0?=w366:bool)
                    n207 = Not Equal To 0?(x=w373) -> (x != 0?=w368:bool)
                    n208 = Not Equal To 0?(x=w374) -> (x != 0?=w370:bool)
                    n209 = Not Equal To 0?(x=w376) -> (x != 0?=w375:bool)
                    n210 = Not Equal To 0?(x=w379) -> (x != 0?=w378:bool)
                    n211 = case shown="真" w381 {
                      tunnel: [_ w413] -> w380
                      tunnel: w383 -> [_ w412]
                      frame False {
                      }
                      frame True {
                        n212 = call "获取最近两组水样测试数据.vi"("error in (no error)"=w412, "table"="pH") -> ("error out"=w416:errorcluster, "存储变量"=w415:T14)  [unwired: 8 in]
                        n213 = call "集成干预测试数据存储.vi"("error in (no error)"=w416, "存储变量"=w415) -> ("error out"=w413:errorcluster)  [unwired: 9 in]
                      }
                    }
                    n214 = case shown="真" w378 {
                      tunnel: [_ w408] -> w377
                      tunnel: w380 -> [_ w407]
                      frame False {
                      }
                      frame True {
                        n215 = call "获取最近两组水样测试数据.vi"("error in (no error)"=w407, "table"="DO") -> ("error out"=w411:errorcluster, "存储变量"=w410:T14)  [unwired: 8 in]
                        n216 = call "集成干预测试数据存储.vi"("error in (no error)"=w411, "存储变量"=w410) -> ("error out"=w408:errorcluster)  [unwired: 9 in]
                      }
                    }
                    n217 = case shown="真" w375 {
                      tunnel: [_ w403] -> w371
                      tunnel: w377 -> [_ w402]
                      frame False {
                      }
                      frame True {
                        n218 = call "获取最近两组水样测试数据.vi"("error in (no error)"=w402, "table"="比电导率") -> ("error out"=w406:errorcluster, "存储变量"=w405:T14)  [unwired: 8 in]
                        n219 = call "集成干预测试数据存储.vi"("error in (no error)"=w406, "存储变量"=w405) -> ("error out"=w403:errorcluster)  [unwired: 9 in]
                      }
                    }
                    n220 = case shown="真" w370 {
                      tunnel: [_ w398] -> w369
                      tunnel: w371 -> [_ w397]
                      frame False {
                      }
                      frame True {
                        n221 = call "获取最近两组水样测试数据.vi"("error in (no error)"=w397, "table"="浊度") -> ("error out"=w401:errorcluster, "存储变量"=w400:T14)  [unwired: 8 in]
                        n222 = call "集成干预测试数据存储.vi"("error in (no error)"=w401, "存储变量"=w400) -> ("error out"=w398:errorcluster)  [unwired: 9 in]
                      }
                    }
                    n223 = case shown="真" w368 {
                      tunnel: [_ w393] -> w367
                      tunnel: w369 -> [_ w392]
                      frame False {
                      }
                      frame True {
                        n224 = call "获取最近两组水样测试数据.vi"("error in (no error)"=w392, "table"="叶绿素") -> ("error out"=w396:errorcluster, "存储变量"=w395:T14)  [unwired: 8 in]
                        n225 = call "集成干预测试数据存储.vi"("error in (no error)"=w396, "存储变量"=w395) -> ("error out"=w393:errorcluster)  [unwired: 9 in]
                      }
                    }
                    n226 = case shown="真" w366 {
                      tunnel: [_ w388] -> _
                      tunnel: w367 -> [_ w387]
                      frame False {
                      }
                      frame True {
                        n227 = call "获取最近两组水样测试数据.vi"("error in (no error)"=w387, "table"="藻密度") -> ("error out"=w391:errorcluster, "存储变量"=w390:T14)  [unwired: 8 in]
                        n228 = call "集成干预测试数据存储.vi"("error in (no error)"=w391, "存储变量"=w390) -> ("error out"=w388:errorcluster)  [unwired: 9 in]
                      }
                    }
                  }
                }
              }
            }
          }
        }
        n229 = global read "采配水全局变量.vi" "状态"() -> (w267:T10)
        n230 = Unbundle By Name(w267) -> ("R0"=w266:i16)
        n231 = Equal To 0?(x=w266) -> (x = 0?=w265:bool)
        n232 = Select(t=enum16{"初始化", "采配水启动", "仪器操作", "反冲洗", "结束"}."结束" ("枚举"), s=w265, f=enum16{"初始化", "采配水启动", "仪器操作", "反冲洗", "结束"}."反冲洗" ("枚举")) -> (s? t:f=w262:enum16{"初始化", "采配水启动", "仪器操作", "反冲洗", "结束"})
      }
      frame "结束" {
        n233 = Release Queue(queue=w438) -> ()  [unwired: 2 in, 3 out]
        n234 = Unbundle By Name(w435) -> ("测试模式"=w436:enum16{"正常测试", "集成干预"})
        n235 = Cancel Notification(0:w439) -> (8:w440:refnum<notifier>)  [unwired: 1 in, 2 out]
        n236 = Release Notifier(notifier=w440) -> ()  [unwired: 2 in, 3 out]
        n237 = case shown="\"集成干预\"" w436 {
          tunnel: w434 -> [_ w443]
          frame "正常测试", Default {
          }
          frame "集成干预" {
            n238 = global write "系统设置全局变量.vi" "运行模式"(w443) -> ()
          }
        }
      }
    }
    n239 = Format Into String(format string="%s,当前运行时间%d秒" ("格式字符串"), w15, w11) -> (resulting string=w16:string)  [unwired: 2 in, 1 out]
    n240 = global write "采配水全局变量.vi" "运行状态显示"(w16) -> ()
  }
